vi "7.6.vi"() -> ()   [LabVIEW 2017]
panel:
  out "波形图":dbl[][](graph)
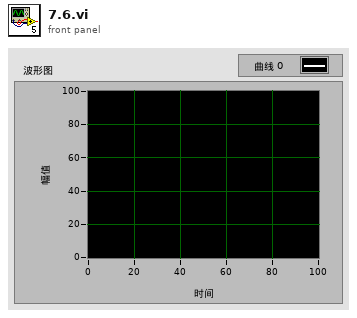
[diagram p1: front panel]
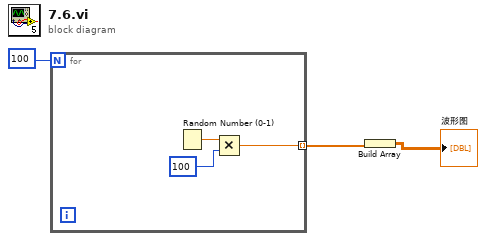
[diagram p0: block diagram]
diagram:
  n1 = for {
    N: 100 -> [_]
    tunnel: [w4] -> w3 mode=indexing
    n2 = Random Number (0-1)() -> (number: 0 to 1=w6:dbl)
    n3 = Multiply(x=w6, y=100) -> (x*y=w4:dbl)
  }
  n4 = Build Array(w3) -> (→"波形图":dbl[][])
